vi "G#100_API_Demo.vi"() -> ()   [LabVIEW 2017, in "G#IDE.lvlib" / "G#100.lvlib"]
doc: "Copyright (c) 2010 AddQ Consulting (www.addq.se). All rights reserved."
uses:
  <resource>/Framework/Providers/AddQ/G#IDE/Providers/G#100.lvlib
  <resource>/Framework/Providers/AddQ/G#IDE/Providers/Provider_G#100/ProviderG#100_class/ClassInfo.ctl
  <resource>/Framework/Providers/AddQ/G#IDE/Providers/Provider_G#100/ProviderG#100_class/MethodInfo.ctl
  <vilib>/LabVIEW Icon API/lv_icon/Classes/Icon/Icon.lvclass
  <resource>/Framework/Providers/AddQ/G#IDE/Providers/Provider_G#100/ProviderG#100_class/ProviderG#100.lvclass
  <resource>/Framework/Providers/AddQ/G#IDE/support/ProviderLib/ProviderLib.lvlib
  <resource>/Framework/Providers/AddQ/G#IDE/support/IconLib/IconLib.lvlib
panel:
  in  "PreDefineClassColors":bool
  out "LVclasspath":path
  out "IconImage":picture
  out "error out":errorcluster
  in  "ControlTypeDefsToCreate":T1[](array[typedef])=[{"MethodName"="MyTypeDef", "MethodPath"=path "", "MethodDescription"="", "Scope"=enum."public", "MethodTemplateName"="", "OpenAfter"=FALSE, "DynamicDispatch"=FALSE, "OverrideMethod"=path "", "Abstract"=FALSE, "Property"=FALSE, "Utils"=FALSE, "Icon"=refnum}]
  in  "MethodsToCreate":T1[](array[typedef])=[{"MethodName"="MyTest", "MethodPath"=path "", "MethodDescription"="", "Scope"=enum."public", "MethodTemplateName"="", "OpenAfter"=TRUE, "DynamicDispatch"=FALSE, "OverrideMethod"=path "", "Abstract"=FALSE, "Property"=FALSE, "Utils"=FALSE, "Icon"=refnum}]
  in  "BodyColor":u32(colorbox)=6618880
  in  "HeaderColor":u32(colorbox)=6735872
  in  "ClassCreationOption":T2={"ClassName"="TestClass", "ClassFolder"=path "F:/tmp/TestClass_class", "ClassDescription"="", "ClassTemplate"="G#Template", "BaseClassPath"=path "", "Abstract"=FALSE}
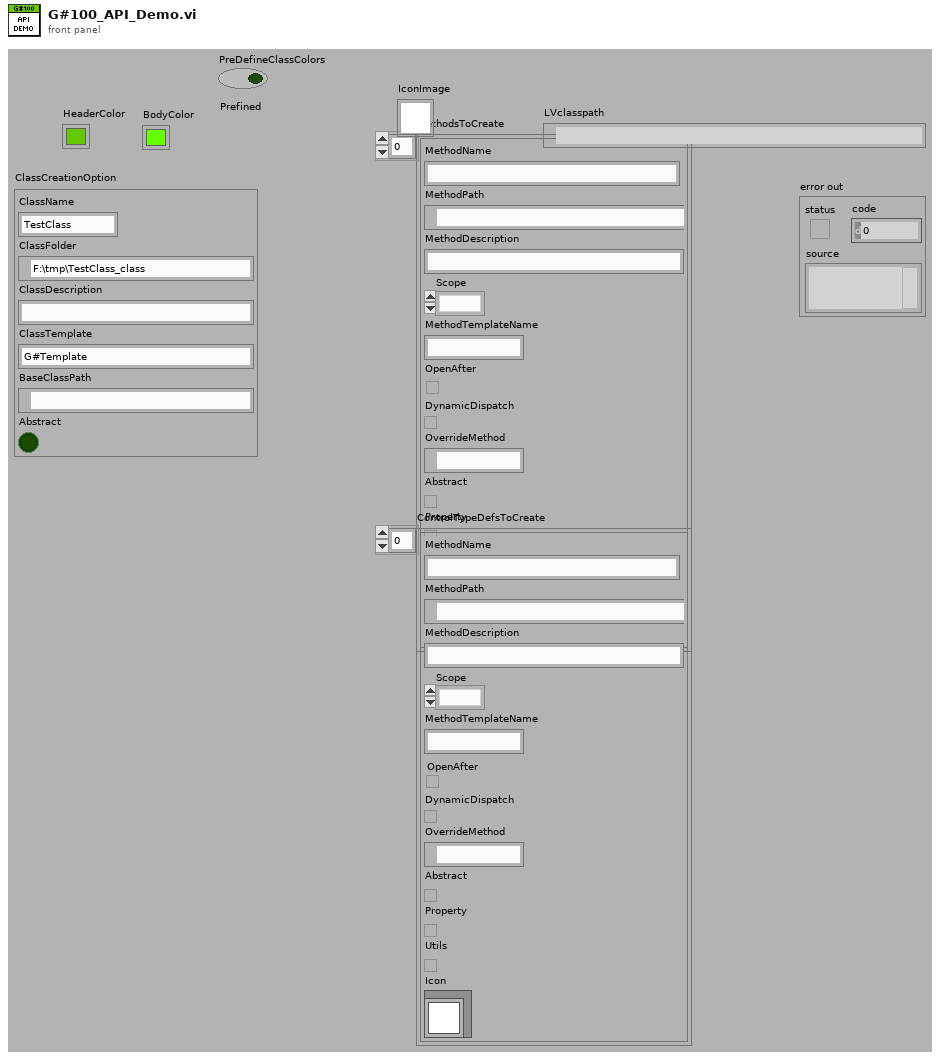
[diagram p1: front panel]
types:
  T1 = typedef "G#IDE.lvlib/ProviderG#100.lvclass/MethodInfo.ctl" = cluster{"MethodName":string, "MethodPath":path, "MethodDescription":string, "Scope":enum32{"invalid scope", "public", "private", "protected", "community"}, "MethodTemplateName":string, "OpenAfter":bool, "DynamicDispatch":bool, "OverrideMethod":path, "Abstract":bool, "Property":bool, "Utils":bool, "Icon":refnum<class "Icon.lvclass">}
  T2 = typedef "G#IDE.lvlib/ProviderG#100.lvclass/ClassInfo.ctl" = cluster{"ClassName":string, "ClassFolder":path, "ClassDescription":string, "ClassTemplate":string, "BaseClassPath":path, "Abstract":bool}
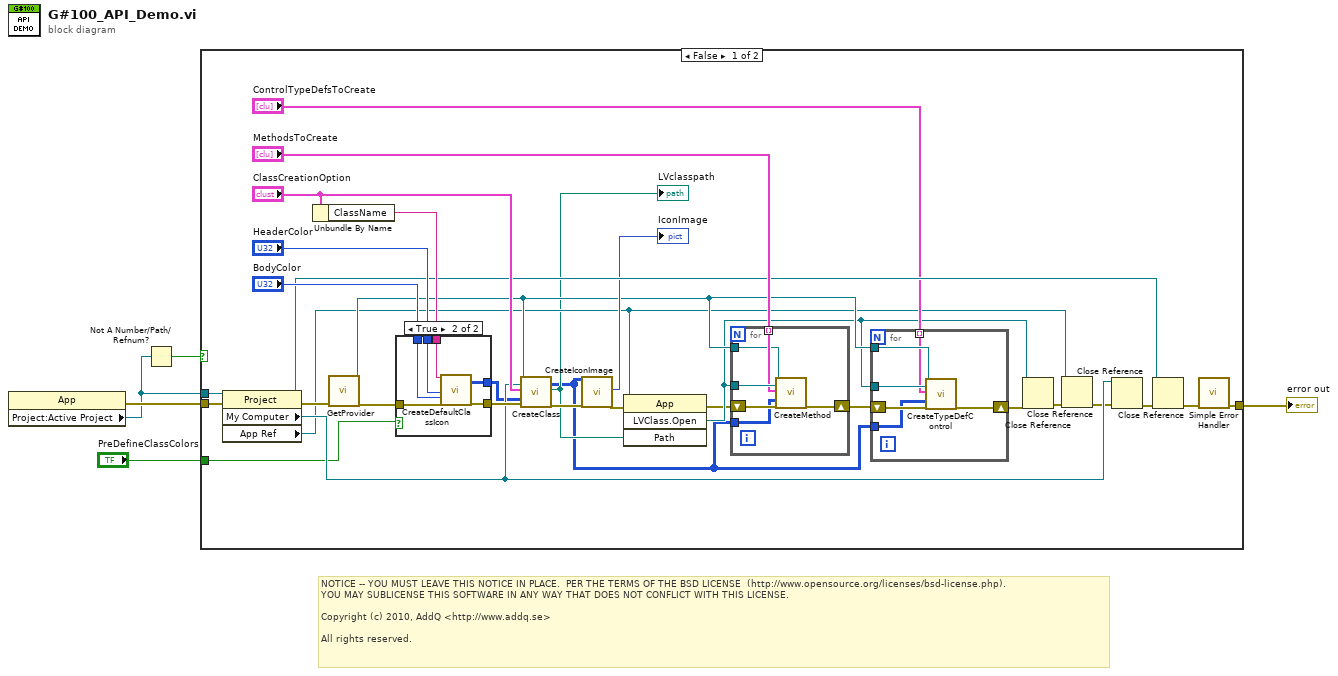
[diagram p0: block diagram]
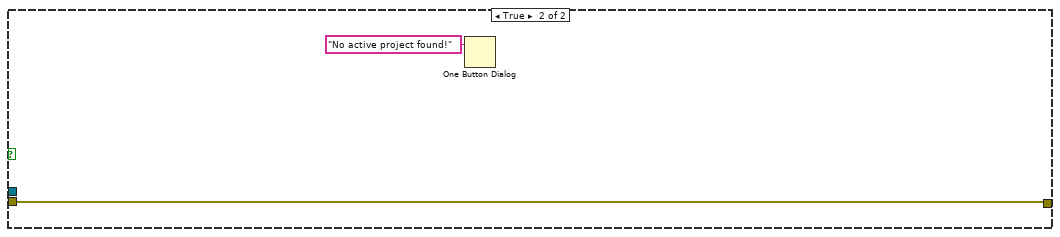
[diagram p3: hidden frame]
diagram:
  # "NOTICE -- YOU MUST LEAVE THIS NOTICE IN PLACE.  PER THE TERMS OF THE BSD LICENSE  (http://www.opensource.org/licenses/bsd-license.php).\nYOU MAY SUBLICENSE THIS SOFTWARE IN ANY WAY THAT DOES NOT CONFLICT WITH THIS LICENSE.\n\nCopyright (c) 2010, AddQ <http://www.addq.se>\n\nAll rights reserved."
  n1 = property class="App"() -> (error out=w2:errorcluster, "Project:Active Project"=w1:refnum<vi>)  [unwired: 2 in, 1 out]
  n2 = Not A Number/Path/Refnum?(number/path/refnum=w1) -> (NaN/Path/Refnum?=w4:bool)
  n3 = case shown="False" w4 {
    tunnel: w2 -> [w36 w57]
    tunnel: [w19 w57] -> w5
    tunnel: w1 -> [w16 _]
    tunnel: "PreDefineClassColors" -> [w14 _]
    frame False {
      n4 = property class="Project"(reference=w16, error in=w36) -> (reference out=w27:refnum<vi>, error out=w29:errorcluster, "My Computer"=w25:refnum<vi>, "App Ref"=w10:refnum<vi>)
      n5 = Unbundle By Name("ClassCreationOption") -> ("ClassName"=w32:string)
      n6 = call <resource>:"GetProvider.vi"("error in (no error)"=w29) -> ("Provider"=w15:refnum<class "ProviderG#100.lvclass">, "error out"=w35:errorcluster)  [unwired: 17 in]
      n7 = case shown="True" w14 {
        tunnel: w35 -> [w37 w43]
        tunnel: [w37 w42] -> w34
        tunnel: w32 -> [_ w38]
        tunnel: "HeaderColor" -> [_ w41]
        tunnel: "BodyColor" -> [_ w40]
        tunnel: [_ w39] -> w23
        frame False {
          # "Force editor\nto popup"
        }
        frame True {
          n8 = call <resource>:"CreateDefaultClassIcon.vi"("HeaderText"=w38, "HeaderColor"=w41, "BodyColor"=w40, "error in (no error)"=w43) -> ("IconOut"=w39:u32[][], "error out"=w42:errorcluster)  [unwired: 14 in]
        }
      }
      n9 = call-dynamic "CreateClass.vi"("ref in"=w15, "ProjectItem"=w25, "ClassInfo"="ClassCreationOption", "IconTemplate"=w23, "error in (no error)"=w34) -> ("ClassIcon"=w6:u32[][], "LVClassPath"=w9:path, "error out"=w18:errorcluster)  [unwired: 11 in, 1 out]
      "LVclasspath" <- w9
      n10 = call <resource>:"CreateIconImage.vi"("Icon"=w6, "error in (no error)"=w18) -> ("IconImage"=→"IconImage":picture, "error out"=w11:errorcluster)  [unwired: 15 in, 1 out]
      n11 = invoke class="App" method="LVClass.Open"(reference=w10, error in=w11, "Path"=w9) -> (error out=w7:errorcluster, "LVClass.Open"=w8:refnum<vi>)  [unwired: 1 in, 2 out]
      n12 = for {
        shift-right: [w54] -> w24
        shift-left: w7 -> [w55]
        tunnel: w15 -> [w50]
        tunnel: w8 -> [w53]
        tunnel: "MethodsToCreate" -> [w52] mode=indexing
        tunnel: w6 -> [w51]
        n13 = call-dynamic "CreateMethod.vi"("ref in"=w50, "LvClassRef"=w53, "MethodInfo"=w52, "IconTemplate"=w51, "error in (no error)"=w55) -> ("error out"=w54:errorcluster)  [unwired: 10 in, 4 out]
      }
      n14 = for {
        shift-right: [w48] -> w21
        shift-left: w24 -> [w49]
        tunnel: w15 -> [w47]
        tunnel: w8 -> [w46]
        tunnel: w6 -> [w45]
        tunnel: "ControlTypeDefsToCreate" -> [w44] mode=indexing
        n15 = call-dynamic "CreateTypeDefControl.vi"("ref in"=w47, "ClassItem"=w46, "ControlData"=w44, "IconTemplate"=w45, "error in (no error)"=w49) -> ("error out"=w48:errorcluster)  [unwired: 11 in, 3 out]
      }
      n16 = Close Reference(reference=w8, error in (no error)=w21) -> (error out=w13:errorcluster)
      n17 = Close Reference(reference=w10, error in (no error)=w13) -> (error out=w12:errorcluster)
      n18 = Close Reference(reference=w25, error in (no error)=w12) -> (error out=w26:errorcluster)
      n19 = Close Reference(reference=w27, error in (no error)=w26) -> (error out=w20:errorcluster)
      n20 = call <vilib>:"Simple Error Handler.vi"("error in (no error)"=w20) -> ("error out"=w19:errorcluster)  [unwired: 4 in, 4 out]
    }
    frame True {
      n21 = One Button Dialog(message="No active project found!") -> ()  [unwired: 1 in, 1 out]
    }
  }
  "error out" <- w5
